vi "Yscaling.vi"(9 "Current Maxed?":bool, 10 "Y":dbl, 11 "Plane Height":dbl) -> (3 "y scaled":dbl, 4 "Testoutput":dbl)   [LabVIEW 2017]
uses:
  <userlib>/PositionDLL/PositionDLL.lvlib
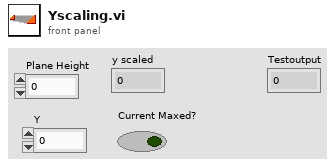
[diagram p1: front panel]
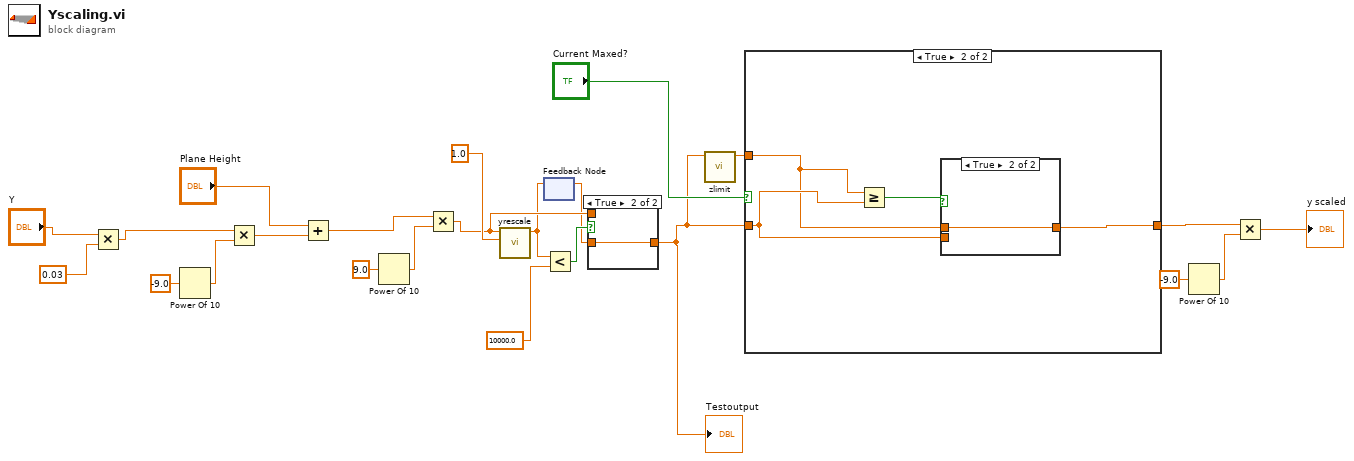
[diagram p0: block diagram]
diagram:
  n1 = Multiply(x="Y", y=0.03) -> (x*y=w19:dbl)
  n2 = Power Of 10(x=-9.0) -> (10^x=w18:dbl)
  n3 = Multiply(x=w19, y=w18) -> (x*y=w20:dbl)
  n4 = Add(x="Plane Height", y=w20) -> (x+y=w23:dbl)
  n5 = Power Of 10(x=9.0) -> (10^x=w22:dbl)
  n6 = Multiply(x=w23, y=w22) -> (x*y=w3:dbl)
  n7 = call <userlib>:"yrescale.vi"("scalingfactor"=1.0, "ylabview"=w3) -> ("function return"=w2:dbl)  [unwired: 9 in]
  n8 = feedback-in #1(w2) -> ()
  n9 = feedback #1() -> (w1:dbl)  [unwired: 1 in]
  n10 = Less?(x=w2, y=10000.0) -> (x < y?=w4:bool)
  n11 = case shown="True" w4 {
    tunnel: [w24 w25] -> w6
    tunnel: w1 -> [_ w25]
    tunnel: w3 -> [w24 _]
    frame False {
    }
    frame True {
    }
  }
  "Testoutput" <- w6
  n12 = call <userlib>:"zlimit.vi"("yscaledinput"=w6) -> ("function return"=w7:dbl)  [unwired: 10 in]
  n13 = case shown="True" "Current Maxed?" {
    tunnel: [w26 w30] -> w8
    tunnel: w6 -> [w26 w28]
    tunnel: w7 -> [_ w27]
    frame False {
    }
    frame True {
      n14 = Greater Or Equal?(x=w27, y=w28) -> (x >= y?=w29:bool)
      n15 = case shown="True" w29 {
        tunnel: w27 -> [_ w32]
        tunnel: [w31 w32] -> w30
        tunnel: w28 -> [w31 _]
        frame False {
        }
        frame True {
        }
      }
    }
  }
  n16 = Power Of 10(x=-9.0) -> (10^x=w11:dbl)
  n17 = Multiply(x=w8, y=w11) -> (x*y=→"y scaled":dbl)
